vi "Test OAuth2.vi"() -> ()   [LabVIEW 2020]
uses:
  OAuth2/Client/Client.lvclass
  OAuth2/Request/Request.lvclass
  OAuth2/OAuth2/OAuth2.lvclass
  OAuth2/Async Authorization/Async Authorization.lvclass
  OAuth2/Authorization/Authorization.lvclass
  OAuth2/Async Auth State.ctl
  OAuth2/OAuth2.lvlib
  OAuth2/Expiry.ctl
panel:
  out "Expiry":T1
  out "error out":errorcluster
  out "State":T2
  in  "Scopes":string[](array[string])
  in  "Redirect URL":string
  in  "Token URL":string
  in  "Auth URL":string
  in  "Client Secret":string
  in  "Client ID":string
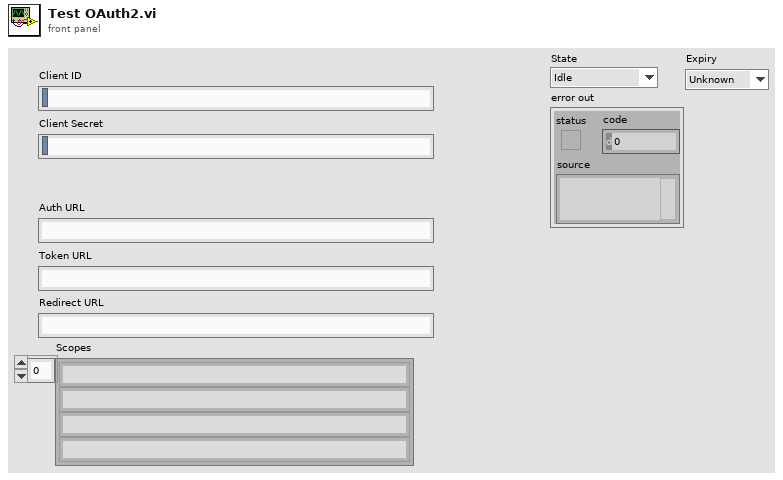
[diagram p1: front panel]
types:
  T1 = typedef "OAuth2.lvlib/Expiry.ctl" = enum16{"Unknown", "Expired", "Good"}
  T2 = typedef "OAuth2.lvlib/Async Auth State.ctl" = enum16{"Idle", "Request", "WaitAuth", "GetToken", "RefreshToken", "Complete", "Failed"}
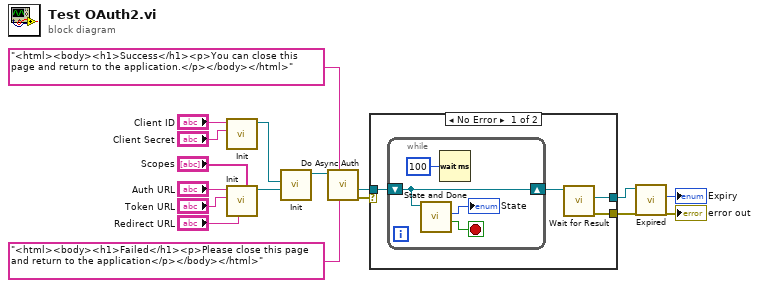
[diagram p0: block diagram]
diagram:
  n1 = call "Init.vi"("Secret"="Client Secret", "ID"="Client ID") -> ("Client out"=w6:refnum<class "Client.lvclass">)  [unwired: 9 in]
  n2 = call "Init.vi"("Scopes"="Scopes", "Redirect URL (http://localhost)"="Redirect URL", "Token URL"="Token URL", "Auth URL"="Auth URL") -> ("Request out"=w7:refnum<class "Request.lvclass">)  [unwired: 7 in]
  n3 = call "Init.vi"("Request"=w7, "Client"=w6) -> ("OAuth2"=w13:refnum<class "OAuth2.lvclass">)  [unwired: 9 in]
  n4 = call "Do Async Auth.vi"("Failed HTML Response"="<html><body><h1>Failed</h1><p>Please close this page and return to the application</p></body></html>" ("Complete Response Content"), "Success HTML Response"="<html><body><h1>Success</h1><p>You can close this page and return to the application.</p></body></html>" ("Complete Response Content"), "OAuth2 in"=w13) -> ("error out"=w10:errorcluster, "Async Authentication"=w12:refnum<class "Async Authorization.lvclass">)  [unwired: 6 in, 1 out]
  n5 = case shown="No Error" w10 {
    selector: w10 -> [_ w25]
    tunnel: w12 -> [w20 _]
    tunnel: [w18 w25] -> w11
    tunnel: [w17 _] -> w9
    frame No Error {
      n6 = while {
        shift-right: [w22] -> w19
        shift-left: w20 -> [w22]
        stop <- w24 stop-if-true
        n7 = call "State and Done.vi"("Async Authorization in"=w22) -> ("Done?"=w24:bool, "State"=→"State":T2)  [unwired: 9 in]
        n8 = Wait (ms)(milliseconds to wait=u32 100) -> ()  [unwired: 1 out]
      }
      n9 = call "Wait for Result.vi"("Async Authorization in"=w19) -> ("error out"=w18:errorcluster, "Authorization"=w17:refnum<class "Authorization.lvclass">)  [unwired: 8 in, 1 out]
    }
    frame Error {
    }
  }
  "error out" <- w11
  n10 = call "Expired.vi"("Authorization in"=w9) -> ("Expiry"=→"Expiry":T1)  [unwired: 10 in]
